vi "Loop_RoboRio_SEN.vi"() -> ()   [LabVIEW 2017, in "System_Status.lvlib"]
uses:
  System_Status.lvlib
  TypeDef Share All/CLUSTER_RoboRio_Status.ctl
  TypeDef Share All/CLUSTER_RoboRio_Faults.ctl
  TypeDef Share All/CLUSTER_RoboRio_Rails.ctl
  TypeDef Share All/CLUSTER_RoboRio_SingleRail.ctl
  CLUSTER_System_CMD.ctl
  Global Share All/Global_STOP.vi
  Global_CMD.vi
  <vilib>/Rock Robotics/WPI/Power/WPI_Power Get 6Volt Rail Voltage and Current.vi
  <vilib>/Rock Robotics/WPI/Power/WPI_Power Get 5Volt Rail Voltage and Current.vi
  <vilib>/Rock Robotics/WPI/Power/WPI_Power Get 3Volt Rail Voltage and Current.vi
  Global_SEN Write_Data.vi
panel:
  out "Cycle Time (S)":dbl format="%.3g"
  in  "Target Time(ms)":u32=50
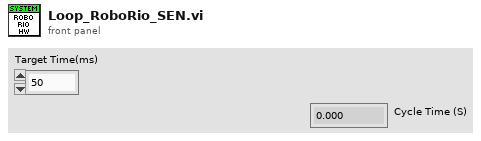
[diagram p1: front panel]
types:
  T1 = typedef "System_Status.lvlib/CLUSTER_System_CMD.ctl" = cluster{"Enable PCM Monitoring":bool, "Enable PDP Monitoring":bool, "Enable RoboRio Monitoring":bool}
  T2 = typedef "CLUSTER_RoboRio_Status.ctl" = cluster{"RoboRio Faults":T3, "RIO inpt vol (V)":dbl, "RIO inpt cur (A)":dbl, "RoboRio Rails":T4}
  T3 = typedef "CLUSTER_RoboRio_Faults.ctl" = cluster{"Inpt. V. Brn. Out":bool, "3.3V Usr Rail Shrt.":bool, "5 V Usr Rail Shrt.":bool, "6 V Usr. Rail Shrt.":bool, "5V Usr. Rail Brn. Out":bool}
  T4 = typedef "CLUSTER_RoboRio_Rails.ctl" = cluster{"3.3 Volt":T5, "5 Volt":T5, "6 Volt":T5}
  T5 = typedef "CLUSTER_RoboRio_SingleRail.ctl" = cluster{"Vol.  (V)":dbl, "Cur. (A)":dbl}
  T6 = cluster{"Target Time(ms)":u32, "Current Time":timestamp, "Previous Time":timestamp, "Cycle Time (S)":dbl, "RoboRio Status":T2, "Enabled":T1}
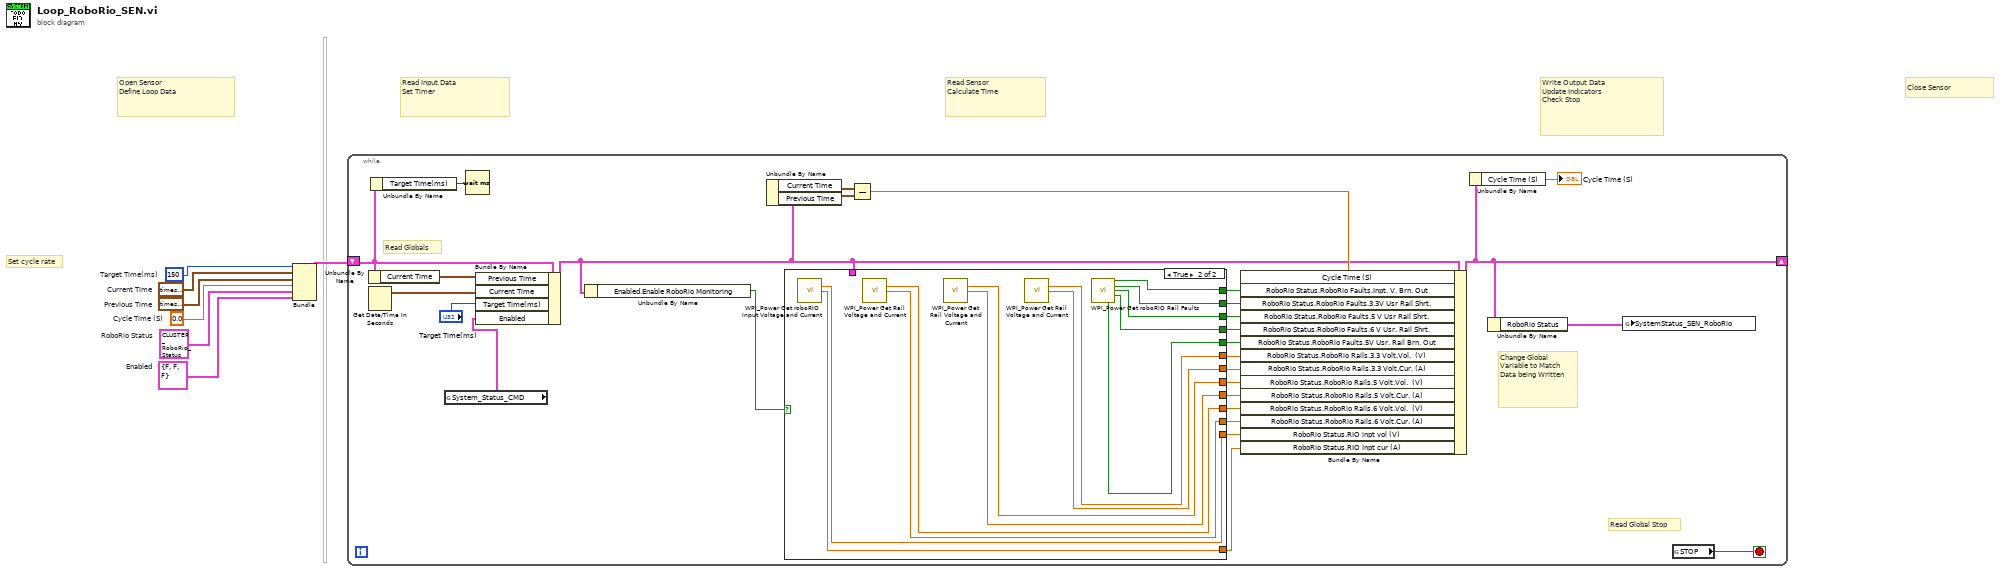
[diagram p0: block diagram]
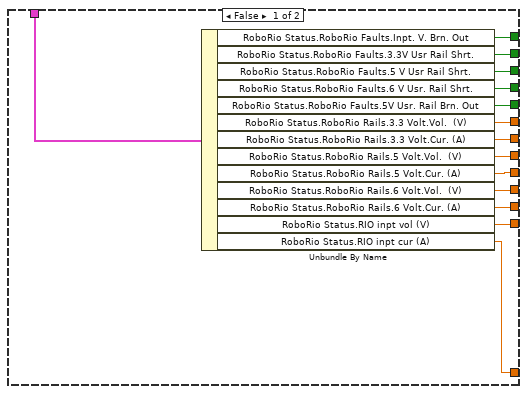
[diagram p2: hidden frame]
diagram:
  w1 = T1 {"Enable PCM Monitoring"=FALSE, "Enable PDP Monitoring"=FALSE, "Enable RoboRio Monitoring"=FALSE}  # Enabled
  w2 = T2 {"RoboRio Faults"={"Inpt. V. Brn. Out"=FALSE, "3.3V Usr Rail Shrt."=FALSE, "5 V Usr Rail Shrt."=FALSE, "6 V Usr. Rail Shrt."=FALSE, "5V Usr. Rail Brn. Out"=FALSE}, "RIO inpt vol (V)"=0.0, "RIO inpt cur (A)"=0.0, "RoboRio Rails"={"3.3 Volt"={"Vol.  (V)"=0.0, "Cur. (A)"=0.0}, "5 Volt"={"Vol.  (V)"=0.0, "Cur. (A)"=0.0}, "6 Volt"={"Vol.  (V)"=0.0, "Cur. (A)"=0.0}}}  # RoboRio Status
  w3 = 0.0  # Cycle Time (S)
  w7 = timestamp(0 s since 1904-01-01)  # Previous Time
  w6 = timestamp(0 s since 1904-01-01)  # Current Time
  w5 = u32 150  # Target Time(ms)
  # "Close Sensor"
  # "Write Output Data\nUpdate Indicators\nCheck Stop"
  # "Read Sensor\nCalculate Time"
  # "Read Input Data\nSet Timer"
  # "Open Sensor\nDefine Loop Data"
  # "Set cycle rate"
  n1 = Bundle("Target Time(ms)"=w5, "Current Time"=w6, "Previous Time"=w7, "Cycle Time (S)"=w3, "RoboRio Status"=w2, "Enabled"=w1) -> (w4:T6)  [unwired: 1 in]
  n2 = while {
    shift-right: [w26] -> _
    shift-left: w4 -> [w28]
    stop <- w35 stop-if-true
    # "Change Global\nVariable to Match\nData being Written"
    # "Read Globals"
    # "Read Global Stop"
    n3 = Unbundle By Name(w28) -> ("Current Time"=w32:timestamp)
    n4 = Get Date/Time In Seconds() -> (seconds since 1Jan1904=w33:timestamp)
    n5 = Unbundle By Name(w28) -> ("Target Time(ms)"=w27:u32)
    n6 = global read "Global_CMD.vi" "System_Status_CMD"() -> (w10:T1)
    n7 = Wait (ms)(milliseconds to wait=w27) -> ()  [unwired: 1 out]
    n8 = Bundle By Name(cluster=w28, "Previous Time"=w32, "Current Time"=w33, "Target Time(ms)"="Target Time(ms)", "Enabled"=w10) -> (w8:T6)
    n9 = Unbundle By Name(w8) -> ("Enabled.Enable RoboRio Monitoring"=w9:bool)
    n10 = Unbundle By Name(w8) -> ("Current Time"=w31:timestamp, "Previous Time"=w30:timestamp)
    n11 = case shown="True" w9 {
      tunnel: [w48 w62] -> w23
      tunnel: [w36 w61] -> w22
      tunnel: [w47 w60] -> w21
      tunnel: [w46 w59] -> w20
      tunnel: [w45 w58] -> w19
      tunnel: [w44 w57] -> w18
      tunnel: [w43 w56] -> w17
      tunnel: [w42 w55] -> w16
      tunnel: [w41 w54] -> w15
      tunnel: [w40 w53] -> w14
      tunnel: [w39 w52] -> w13
      tunnel: [w38 w51] -> w12
      tunnel: [w37 w50] -> w11
      tunnel: w8 -> [w49 _]
      frame False {
        n12 = Unbundle By Name(w49) -> ("RoboRio Status.RoboRio Faults.Inpt. V. Brn. Out"=w37:bool, "RoboRio Status.RoboRio Faults.3.3V Usr Rail Shrt."=w38:bool, "RoboRio Status.RoboRio Faults.5 V Usr Rail Shrt."=w39:bool, "RoboRio Status.RoboRio Faults.6 V Usr. Rail Shrt."=w40:bool, "RoboRio Status.RoboRio Faults.5V Usr. Rail Brn. Out"=w41:bool, "RoboRio Status.RoboRio Rails.3.3 Volt.Vol.  (V)"=w42:dbl, "RoboRio Status.RoboRio Rails.3.3 Volt.Cur. (A)"=w43:dbl, "RoboRio Status.RoboRio Rails.5 Volt.Vol.  (V)"=w44:dbl, "RoboRio Status.RoboRio Rails.5 Volt.Cur. (A)"=w45:dbl, "RoboRio Status.RoboRio Rails.6 Volt.Vol.  (V)"=w46:dbl, "RoboRio Status.RoboRio Rails.6 Volt.Cur. (A)"=w47:dbl, "RoboRio Status.RIO inpt vol (V)"=w48:dbl, "RoboRio Status.RIO inpt cur (A)"=w36:dbl)
      }
      frame True {
        n13 = call <vilib>:"WPI_Power Get roboRIO Input Voltage and Current.vi"() -> ("roboRIO input voltage (V)"=w62:dbl, "roboRIO input current (A)"=w61:dbl)  [unwired: 13 in, 1 out]
        n14 = call-poly <vilib>:"WPI_Power Get Rail Voltage and Current.vi"() -> ("6 volt rail voltage (V)"=w59:dbl, "6 volt rail current (A)"=w60:dbl)  [unwired: 13 in, 1 out]
        n15 = call-poly <vilib>:"WPI_Power Get Rail Voltage and Current.vi"() -> ("5 volt rail voltage (V)"=w57:dbl, "5 volt rail current (A)"=w58:dbl)  [unwired: 13 in, 1 out]
        n16 = call-poly <vilib>:"WPI_Power Get Rail Voltage and Current.vi"() -> ("3.3 volt rail voltage (V)"=w55:dbl, "3.3 volt rail current (A)"=w56:dbl)  [unwired: 13 in, 1 out]
        n17 = call <vilib>:"WPI_Power Get roboRIO Rail Faults.vi"() -> ("Input Voltage Brown Out"=w50:bool, "3.3V User Rail Short"=w51:bool, "5 V User Rail Short"=w52:bool, "6 V User Rail Short"=w53:bool, "5V User Rail Brown Out"=w54:bool)  [unwired: 10 in, 1 out]
      }
    }
    n18 = Subtract(x=w31, y=w30) -> (x-y=w24:dbl)
    n19 = Bundle By Name(cluster=w8, "Cycle Time (S)"=w24, "RoboRio Status.RoboRio Faults.Inpt. V. Brn. Out"=w11, "RoboRio Status.RoboRio Faults.3.3V Usr Rail Shrt."=w12, "RoboRio Status.RoboRio Faults.5 V Usr Rail Shrt."=w13, "RoboRio Status.RoboRio Faults.6 V Usr. Rail Shrt."=w14, "RoboRio Status.RoboRio Faults.5V Usr. Rail Brn. Out"=w15, "RoboRio Status.RoboRio Rails.3.3 Volt.Vol.  (V)"=w16, "RoboRio Status.RoboRio Rails.3.3 Volt.Cur. (A)"=w17, "RoboRio Status.RoboRio Rails.5 Volt.Vol.  (V)"=w18, "RoboRio Status.RoboRio Rails.5 Volt.Cur. (A)"=w19, "RoboRio Status.RoboRio Rails.6 Volt.Vol.  (V)"=w20, "RoboRio Status.RoboRio Rails.6 Volt.Cur. (A)"=w21, "RoboRio Status.RIO inpt vol (V)"=w23, "RoboRio Status.RIO inpt cur (A)"=w22) -> (w26:T6)
    n20 = Unbundle By Name(w26) -> ("Cycle Time (S)"=→"Cycle Time (S)":dbl)
    n21 = Unbundle By Name(w26) -> ("RoboRio Status"=w34:T2)
    n22 = global write "Global_SEN Write_Data.vi" "SystemStatus_SEN_RoboRio"(w34) -> ()
    n23 = global read "Global_STOP.vi" "STOP"() -> (w35:bool)
  }
